vi "Gas Menu.vi"(7 "Set? (F:Read)":bool, 8 "Error In":errorcluster, 9 "Gas Menu (0)":i32, 11 "VISA resource name":refnum<visa-resource-name>) -> (0 "Error Out":errorcluster, 1 "Gas Menu out":i32, 3 "dup VISA resource name":refnum<visa-resource-name>)   [LabVIEW 2016, in "MGC647C.lvlib"]
doc: "Read/set gas menu."
uses:
  MGC647C.lvlib
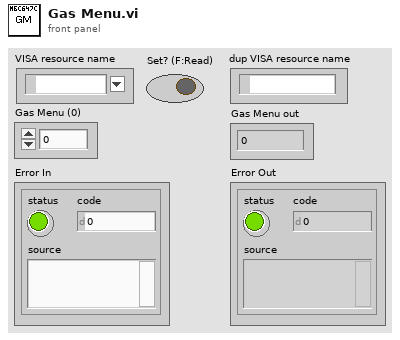
[diagram p1: front panel]
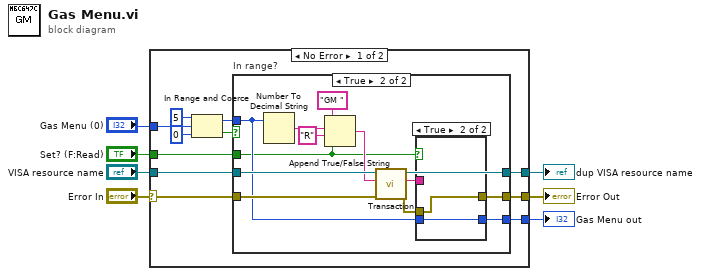
[diagram p0: block diagram]
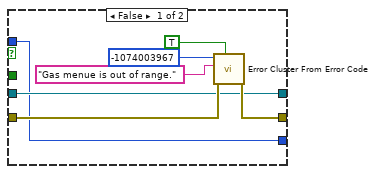
[diagram p2: hidden frame]
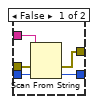
[diagram p3: hidden frame]
diagram:
  n1 = case shown="No Error" "Error In" {
    selector: "Error In" -> [w9 w47]
    tunnel: "VISA resource name" -> [w18 w46]
    tunnel: [w17 w46] -> w6
    tunnel: [w16 w47] -> w5
    tunnel: "Set? (F:Read)" -> [w15 _]
    tunnel: "Gas Menu (0)" -> [w14 w48]
    tunnel: [w8 w48] -> w1
    frame No Error {
      n2 = In Range and Coerce(upper limit=5, x=w14, lower limit=0) -> (coerced(x)=w13:i32, In Range?=w10:bool)
      n3 = case "In range?" shown="True" w10 {
        tunnel: w18 -> [w23 w38]
        tunnel: [w23 w37] -> w17
        tunnel: [w24 w32] -> w16
        tunnel: w15 -> [_ w26]
        tunnel: w13 -> [w19 w28]
        tunnel: w9 -> [w25 w29]
        tunnel: [w19 w31] -> w8
        frame False {
          n4 = call <vilib>:"Error Cluster From Error Code.vi"("show call chain? (False)"=TRUE, "error in (no error)"=w25, "error message (\"\")"="Gas menue is out of range." ("error message (\"\")"), "error code (0)"=-1074003967) -> ("error out"=w24:errorcluster)  [unwired: 5 in]
        }
        frame True {
          n5 = Number To Decimal String(number=w28) -> (decimal integer string=w27:string)  [unwired: 1 in]
          n6 = Append True/False String(1:w26, 2:"R" ("false string"), 3:w27, 4:"GM " ("string (\"\")")) -> (0:w30:string)
          n7 = call "Transaction.vi"("Error In"=w29, "Command"=w30, "VISA resource name"=w38) -> ("Error Out"=w33:errorcluster, "Response"=w34:string, "dup VISA resource name"=w37:refnum<visa-resource-name>)  [unwired: 6 in]
          n8 = case shown="True" w26 {
            tunnel: w34 -> [w43 _]
            tunnel: w33 -> [w42 w45]
            tunnel: [w41 w45] -> w32
            tunnel: [w40 w44] -> w31
            tunnel: w28 -> [w39 w44]
            frame False {
              n9 = Scan From String(input string=w43, error in=w42, default 1=w39) -> (error out=w41:errorcluster, output 1=w40:i32)  [unwired: 2 in, 2 out]
            }
            frame True {
            }
          }
        }
      }
    }
    frame Error {
    }
  }
  "dup VISA resource name" <- w6
  "Error Out" <- w5
  "Gas Menu out" <- w1
